vi "FPGA_PPG_load.vi"(0 "resource_in":refnum<visa-resource-name>, 2 "command_lines":string[](array[string]), 5 "error in (no error)":errorcluster) -> (14 "resource_out":refnum<visa-resource-name>, 19 "error out":errorcluster)   [LabVIEW 2014, in "NI-FPGA_PPG_Driver.lvlib"]
doc: "Loads the complete command sequence to the FPGA target.\n\nContact: Falk Ziegler, eMail: ziegler@physik.uni-greifswald.de"
uses:
  NI-FPGA_PPG_Driver.lvlib
  <vilib>/rvi/interface/nirviReadWriteControl/nirviReadWriteControl.xnode
  <vilib>/rvi/interface/nirviMethod/nirviMethod.xnode
  FPGA_PPG_action_type.ctl
  FPGA_PPG_error_type.ctl
  <vilib>/rvi/errors/niLvFpgaAdjustHostInterfaceError.vi
  FPGA_PPG_vi_ref.ctl
  FPGA Bitfiles/TiTaProj_COF_PPG_100MHz.lvbitx
  <vilib>/rvi/errors/niLvFpgaMergeErrorWithErrorCode.vi
  <vilib>/FPGAPlugInAG/PXI-7852R/niLvFpga_WriteFifo_PXI-7852R.vi
panel:
  in  "errorCodes":T1=enum."can't change state while pattern output is in progress"
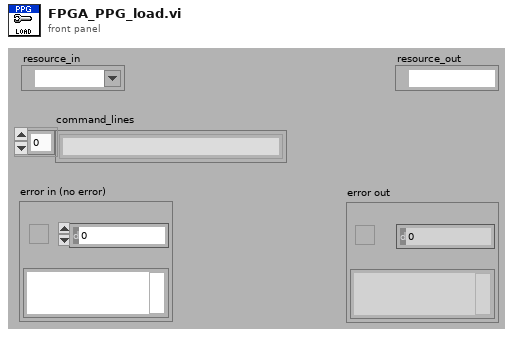
[diagram p1: front panel]
types:
  T1 = typedef "NI-FPGA_PPG_Driver.lvlib/FPGA_PPG_error_type.ctl" = enum16{"no error", "resource not initialized (no commands and invalid mem address)", "wrong memory address (address > Nof commands)", "invalid time value (probably too short)", "cannot start FPGA because one or more errors occured", "FIFO (internal) empty unexpectedly", "DMA FIFO (download from host) full unexpectedly", "checking number of commands: failed", "unknown error 8", "unknown error 9", "unknown error 10", "unknown error 11", "unknown error 12", "unknown error 13", "unknown error 14", "unknown error 15", "unknown error 16", "unknown error 17", "unknown error 18", "unknown error 19", "can't change state while pattern output is in progress"}
  T2 = typedef "NI-FPGA_PPG_Driver.lvlib/FPGA_PPG_action_type.ctl" = enum16{"GET", "SET", "REMOVE"}
  T3 = typedef "NI-FPGA_PPG_Driver.lvlib/FPGA_PPG_vi_ref.ctl" = refnum<k20>
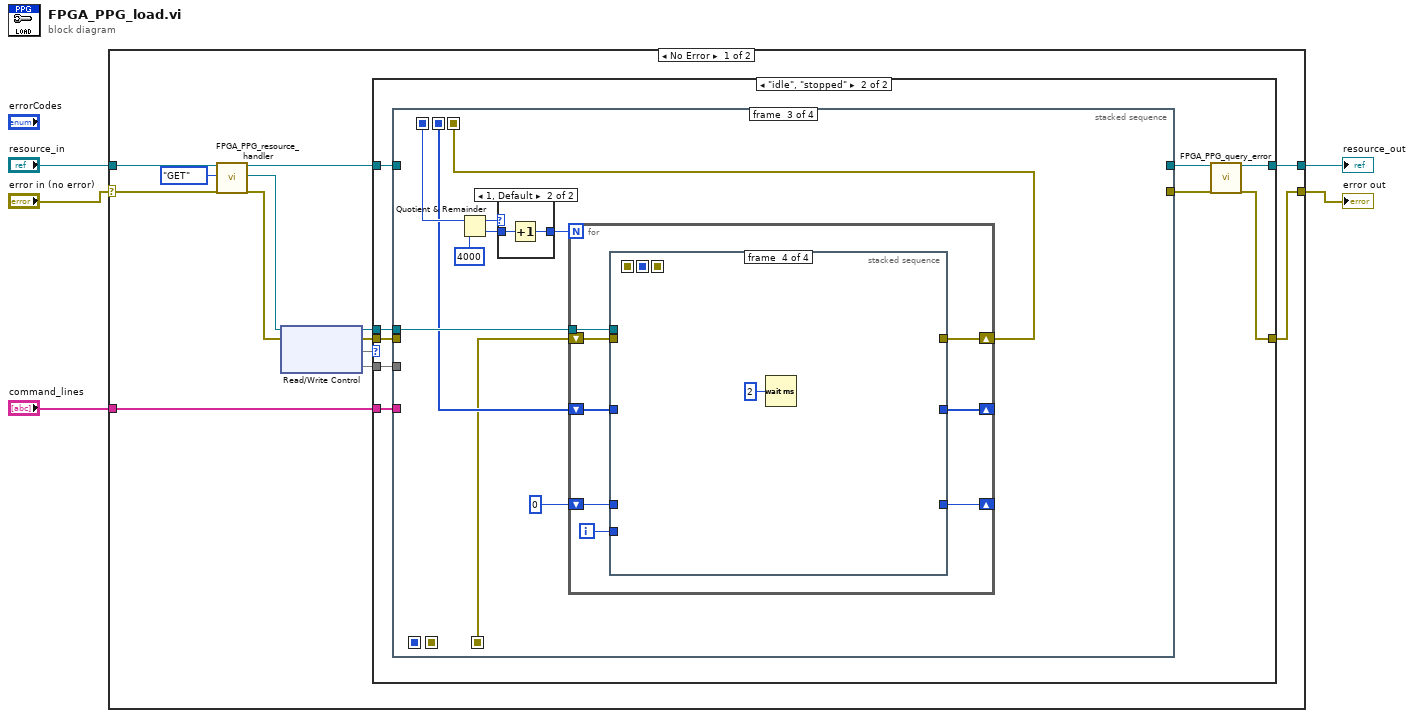
[diagram p0: block diagram]
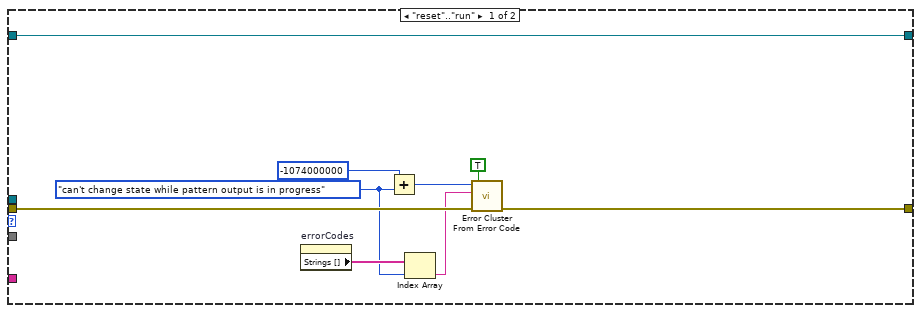
[diagram p2: hidden frame]
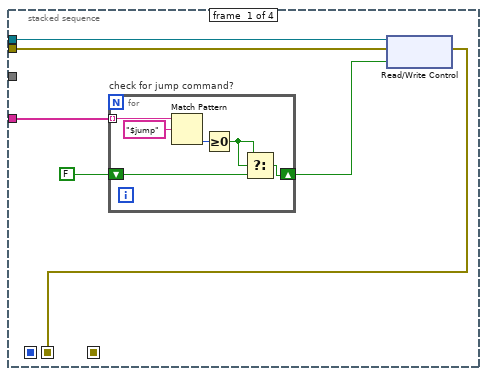
[diagram p3: hidden frame]
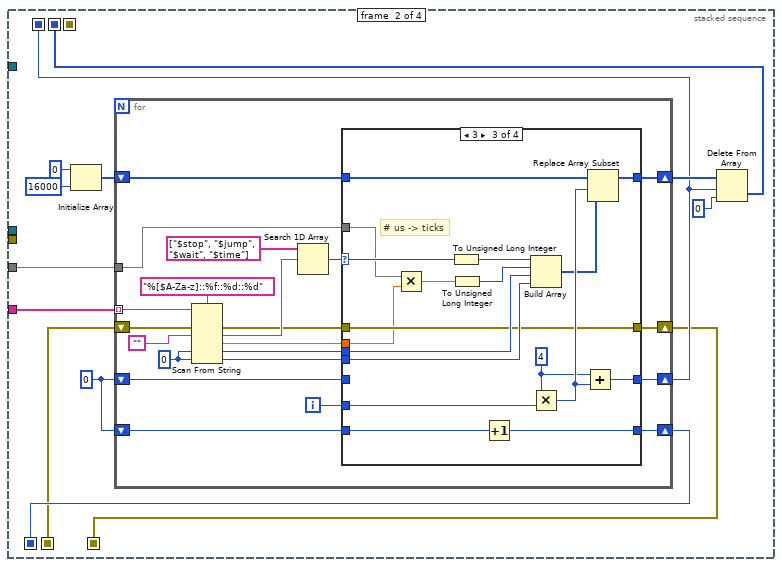
[diagram p4: hidden frame]
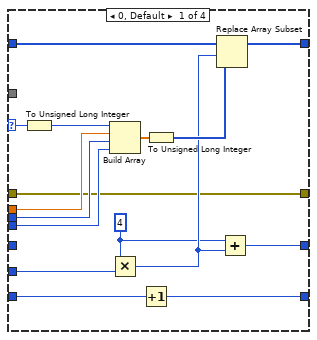
[diagram p5: hidden frame]
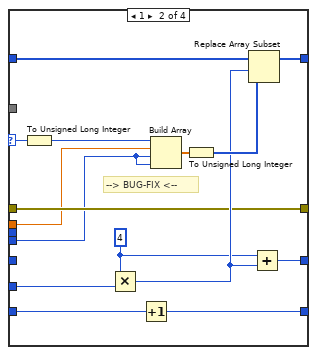
[diagram p6: hidden frame]
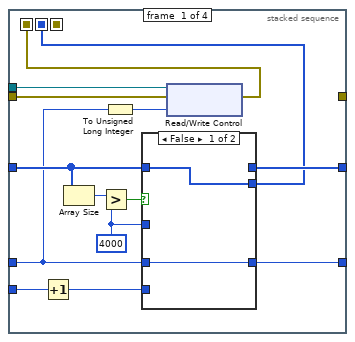
[diagram p9: hidden frame]
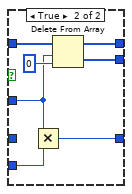
[diagram p10: hidden frame]
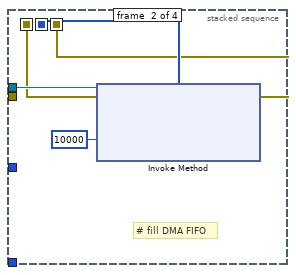
[diagram p11: hidden frame]
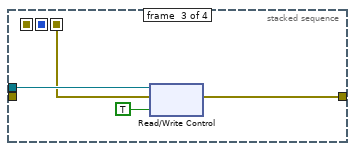
[diagram p12: hidden frame]
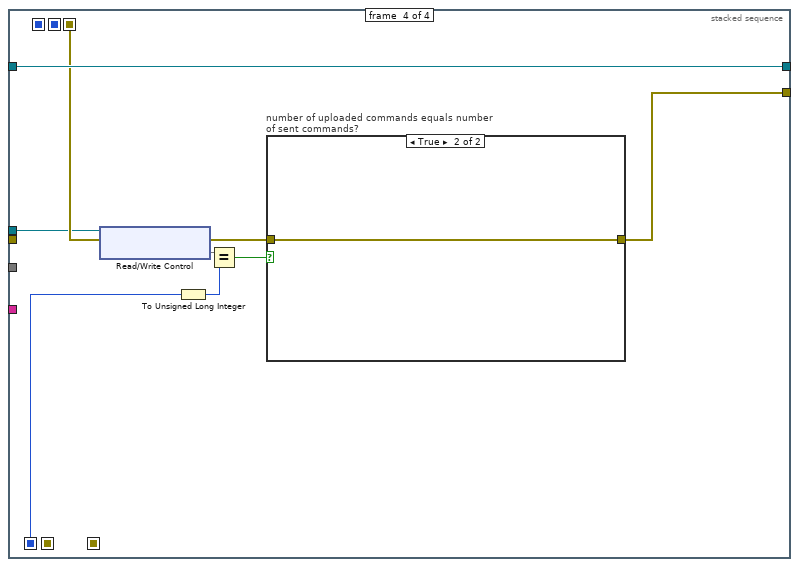
[diagram p13: hidden frame]
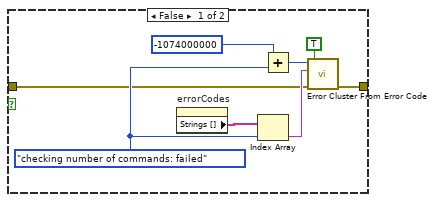
[diagram p14: hidden frame]
diagram:
  n1 = case shown="No Error" "error in (no error)" {
    selector: "error in (no error)" -> [w17 w209]
    tunnel: [w11 w209] -> w4
    tunnel: [w10 w208] -> w3
    tunnel: "resource_in" -> [w18 w208]
    tunnel: "command_lines" -> [w6 _]
    frame No Error {
      n2 = call "FPGA_PPG_resource_handler.vi"("resource_in"=w18, "action"=FPGA_PPG_action_type."GET", "error in (no error)"=w17) -> ("resource_out"=w16:refnum<visa-resource-name>, "FPGA VI Reference Out"=w8:T3, "error out"=w13:errorcluster)  [unwired: 14 in]
      n3 = xnode "Read/Write Control"("FPGA VI Reference In"=w8, "error in"=w13) -> ("FPGA VI Reference Out"=w15:T3, "error out"=w14:errorcluster, "state"=w12, "ticks_per_us"=w7)
      n4 = case shown="\"idle\", \"stopped\"" w12 {
        tunnel: w16 -> [w27 w36]
        tunnel: [w27 w29] -> w10
        tunnel: w6 -> [_ w35]
        tunnel: w15 -> [_ w34]
        tunnel: w14 -> [w26 w33]
        tunnel: [w24 w30] -> w11
        tunnel: w7 -> [_ w28]
        frame "reset".."run" {
          w19 = FPGA_PPG_error_type."can't change state while pattern output is in progress" ("error code (0)")
          n5 = property on="errorCodes" class="Enum (strict)"() -> ("Strings []"=w23:string[])  [unwired: 2 in, 2 out]
          n6 = Add(x=-1074000000 ("error code (0)"), y=w19) -> (x+y=w20:i32)
          n7 = Index Array(array=w23, index=w19) -> (element=w22:string)
          n8 = call <vilib>:"Error Cluster From Error Code.vi"("show call chain? (False)"=TRUE, "error in (no error)"=w26, "error message (\"\")"=w22, "error code (0)"=w20) -> ("error out"=w24:errorcluster)  [unwired: 5 in]
        }
        frame "idle", "stopped" {
          n9 = stacked-sequence {
            seq-local: [_ w56 _ _] -> [_ _ w139 _]
            seq-local: [_ w55 _ _] -> [_ _ w143 _]
            seq-local: [_ _ w137 _] -> [_ _ _ w197]
            seq-local: [_ w53 _ _] -> [_ _ _ w190]
            seq-local: [_ w51 _ _] -> [_ _ w136 _]
            seq-local: [w37 _ _ _] -> [_ w49 _ _]
            tunnel: w34 -> [w40 _ w145 w196]
            tunnel: w36 -> [_ _ _ w198]
            tunnel: [_ _ _ w198] -> w32
            tunnel: w33 -> [w39 _ _ _]
            tunnel: w35 -> [w42 w61 _ _]
            tunnel: [_ _ _ w191] -> w31
            tunnel: w28 -> [_ w50 _ _]
            frame #0 {
              n10 = for "check for jump command?" {
                tunnel: w42 -> [w48] mode=indexing
                shift-right: [w44] -> w38
                shift-left: FALSE -> [w43]
                n11 = Match Pattern(string=w48, regular expression="$jump") -> (offset past match=w46:i32)  [unwired: 1 in, 3 out]
                n12 = Greater Or Equal To 0?(x=w46) -> (x >= 0?=w45:bool)
                n13 = Select(t=w45, s=w45, f=w43) -> (s? t:f=w44:bool)
              }
              n14 = xnode "Read/Write Control"("FPGA VI Reference In"=w40, "error in"=w39, "useJump"=w38) -> ("error out"=w37:errorcluster)  [unwired: 1 out]
            }
            frame #1 {
              w54 = 0
              n15 = Initialize Array(u32 0 ("element"), 16000 ("dimension size")) -> (w60:u32[])
              n16 = for {
                tunnel: w61 -> [w81] mode=indexing
                shift-right: [w73] -> w57
                shift-left: w60 -> [w75]
                shift-right: [w72] -> w55
                shift-left: w54 -> [w71]
                shift-right: [w67] -> w53
                shift-left: w54 -> [w68]
                shift-right: [w65] -> w51
                shift-left: w49 -> [w64]
                tunnel: w50 -> [w62]
                i -> [w74]
                w69 = u32 0
                n17 = Scan From String(format string="%[$A-Za-z]::%f::%d::%d", input string=w81, error in=w64, default 1="" ("default value 1"), default 3=w69, default 4=w69) -> (error out=w66:errorcluster, output 1=w79:string, output 2=w70:dbl, output 3=w77:u32, output 4=w76:u32)  [unwired: 2 in, 2 out]
                n18 = Search 1D Array(1D array=string[] ["$stop", "$jump", "$wait", "$time"], element=w79) -> (index of element=w78:i32)  [unwired: 1 in]
                n19 = case shown="3" w78 {
                  selector: w78 -> [w85 w103 w117 _]
                  tunnel: w70 -> [w86 w100 w116 _]
                  tunnel: w77 -> [w98 _ w131 _]
                  tunnel: w76 -> [w97 w99 w130 _]
                  tunnel: w75 -> [w95 w112 w128 w135]
                  tunnel: w74 -> [w96 w113 w129 _]
                  tunnel: [w92 w109 w127 w135] -> w73
                  tunnel: [w91 w108 w126 w134] -> w72
                  tunnel: w71 -> [_ _ _ w134]
                  tunnel: w68 -> [w88 w105 w120 w133]
                  tunnel: [w87 w104 w119 w133] -> w67
                  tunnel: w66 -> [w83 w101 w118 w132]
                  tunnel: [w83 w101 w118 w132] -> w65
                  tunnel: w62 -> [_ _ w114 _]
                  frame 0, Default {
                    w89 = 4 ("x")
                    n20 = To Unsigned Long Integer(number=w85) -> (unsigned 32bit integer=w84:u32)
                    n21 = Build Array(w84, w86, w98, w97) -> (w94:dbl[])
                    n22 = Multiply(x=w89, y=w96) -> (x*y=w90:i32)
                    n23 = Increment(x=w88) -> (x+1=w87:i32)
                    n24 = To Unsigned Long Integer(number=w94) -> (unsigned 32bit integer=w93:u32[])
                    n25 = Replace Array Subset(array=w95, new element=w93, index=w90) -> (w92:u32[])
                    n26 = Add(x=w89, y=w90) -> (x+y=w91:i32)
                  }
                  frame 1 {
                    w106 = 4 ("x")
                    # "--> BUG-FIX <--"
                    n27 = To Unsigned Long Integer(number=w103) -> (unsigned 32bit integer=w102:u32)
                    n28 = Multiply(x=w106, y=w113) -> (x*y=w107:i32)
                    n29 = Increment(x=w105) -> (x+1=w104:i32)
                    n30 = Build Array(w102, w100, w99, w99) -> (w111:dbl[])
                    n31 = To Unsigned Long Integer(number=w111) -> (unsigned 32bit integer=w110:u32[])
                    n32 = Replace Array Subset(array=w112, new element=w110, index=w107) -> (w109:u32[])
                    n33 = Add(x=w106, y=w107) -> (x+y=w108:i32)
                  }
                  frame 3 {
                    w124 = 4 ("x")
                    # "# us -> ticks"
                    n34 = Multiply(x=w114, y=w116) -> (x*y=w115:dbl)
                    n35 = To Unsigned Long Integer(number=w117) -> (unsigned 32bit integer=w121:u32)
                    n36 = To Unsigned Long Integer(number=w115) -> (unsigned 32bit integer=w123:u32)
                    n37 = Increment(x=w120) -> (x+1=w119:i32)
                    n38 = Build Array(w121, w123, w131, w130) -> (w122:u32[])
                    n39 = Multiply(x=w124, y=w129) -> (x*y=w125:i32)
                    n40 = Add(x=w124, y=w125) -> (x+y=w126:i32)
                    n41 = Replace Array Subset(array=w128, new element=w122, index=w125) -> (w127:u32[])
                  }
                  frame -1 {
                  }
                }
              }
              n42 = Delete From Array(array=w57, length=w55, index=0) -> (deleted portion=w56:u32[])  [unwired: 1 out]
            }
            frame #2 {
              n43 = Quotient & Remainder(x=w143, y=4000) -> (x-y*floor(x/y)=w141:i32, floor(x/y)=w140:i32)
              n44 = case shown="1, Default" w141 {
                tunnel: w140 -> [w146 w148]
                tunnel: [w146 w147] -> w138
                frame 0 {
                }
                frame 1, Default {
                  n45 = Increment(x=w148) -> (x+1=w147:i32)
                }
              }
              n46 = for {
                N: w138 -> [_]
                shift-right: [w151] -> _
                shift-left: 0 -> [w150]
                shift-right: [w153] -> _
                shift-left: w139 -> [w154]
                shift-right: [w149] -> w137
                shift-left: w136 -> [w155]
                tunnel: w145 -> [w156]
                i -> [w152]
                n47 = stacked-sequence {
                  seq-local: [w158 _ _ _] -> [_ w183 _ _]
                  seq-local: [w157 _ _ _] -> [_ w181 _ _]
                  seq-local: [_ w180 _ _] -> [_ _ w187 _]
                  tunnel: w156 -> [w170 w184 w188 _]
                  tunnel: w155 -> [w169 _ _ _]
                  tunnel: w154 -> [w166 _ _ _]
                  tunnel: [w164 _ _ _] -> w153
                  tunnel: w152 -> [w163 _ _ _]
                  tunnel: [w161 _ _ _] -> w151
                  tunnel: w150 -> [w159 _ _ _]
                  tunnel: [_ _ w185 _] -> w149
                  frame #0 {
                    w165 = 4000 ("y")
                    n48 = Increment(x=w163) -> (x+1=w162:i32)
                    n49 = Array Size(array=w166) -> (size(s)=w168:i32)
                    n50 = Greater?(x=w168, y=w165) -> (0:w167:bool)
                    n51 = To Unsigned Long Integer(number=w159) -> (unsigned 32bit integer=w160:u32)
                    n52 = case shown="False" w167 {
                      tunnel: w166 -> [w172 w179]
                      tunnel: w165 -> [_ w174]
                      tunnel: [_ w177] -> w164
                      tunnel: [w172 w176] -> w158
                      tunnel: w159 -> [w171 _]
                      tunnel: w162 -> [_ w175]
                      tunnel: [w171 w173] -> w161
                      frame False {
                      }
                      frame True {
                        n53 = Multiply(x=w174, y=w175) -> (x*y=w173:i32)
                        n54 = Delete From Array(array=w179, length=w174, index=0) -> (deleted portion=w176:u32[], array with subset deleted=w177:u32[])
                      }
                    }
                    n55 = xnode "Read/Write Control"("FPGA VI Reference In"=w170, "error in"=w169, "mem_addr"=w160) -> ("error out"=w157:errorcluster)  [unwired: 1 out]
                  }
                  frame #1 {
                    # "# fill DMA FIFO"
                    n56 = xnode "Invoke Method"("FPGA VI Reference In"=w184, "error in"=w181, "Data"=w183, "Timeout (ms)"=10000) -> ("error out"=w180:errorcluster)  [unwired: 2 out]
                  }
                  frame #2 {
                    n57 = xnode "Read/Write Control"("FPGA VI Reference In"=w188, "error in"=w187, "load"=TRUE) -> ("error out"=w185:errorcluster)  [unwired: 1 out]
                  }
                  frame #3 {
                    n58 = Wait (ms)(milliseconds to wait=u32 2) -> ()  [unwired: 1 out]
                  }
                }
              }
            }
            frame #3 {
              n59 = xnode "Read/Write Control"("FPGA VI Reference In"=w196, "error in"=w197) -> ("error out"=w192:errorcluster, "number_of_cmds"=w194)  [unwired: 1 out]
              n60 = To Unsigned Long Integer(number=w190) -> (unsigned 32bit integer=w193:u32)
              n61 = Equal?(x=w194, y=w193) -> (x = y?=w195:bool)
              n62 = case "number of uploaded commands equals number of sent commands?" shown="True" w195 {
                tunnel: w192 -> [w199 w207]
                tunnel: [w200 w207] -> w191
                frame False {
                  w206 = FPGA_PPG_error_type."checking number of commands: failed" ("errorCodes")
                  n63 = property on="errorCodes" class="Enum (strict)"() -> ("Strings []"=w202:string[])  [unwired: 2 in, 2 out]
                  n64 = Index Array(array=w202, index=w206) -> (element=w203:string)
                  n65 = Add(x=-1074000000 ("error code (0)"), y=w206) -> (x+y=w205:i32)
                  n66 = call <vilib>:"Error Cluster From Error Code.vi"("show call chain? (False)"=TRUE, "error in (no error)"=w199, "error message (\"\")"=w203, "error code (0)"=w205) -> ("error out"=w200:errorcluster)  [unwired: 5 in]
                }
                frame True {
                }
              }
            }
          }
          n67 = call "FPGA_PPG_query_error.vi"("resource_in"=w32, "error in (no error)"=w31) -> ("resource_out"=w29:refnum<visa-resource-name>, "error out"=w30:errorcluster)  [unwired: 16 in]
        }
      }
    }
    frame Error {
    }
  }
  "error out" <- w4
  "resource_out" <- w3
